vi "String_add_space.vi"(1 "result string in":string) -> (0 "result string out":string)   [LabVIEW 2025]
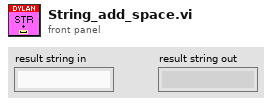
[diagram p1: front panel]
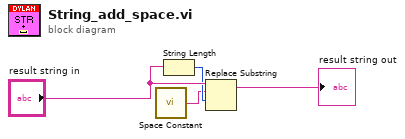
[diagram p0: block diagram]
diagram:
  n1 = call <vilib>:"Space Constant.vi"() -> ("String"=w1:string)
  n2 = String Length(string="result string in") -> (length=w2:i32)
  n3 = Replace Substring(3:w2, 4:w1, 5:"result string in") -> (1:→"result string out":string)  [unwired: 1 in, 1 out]
